vi "SonicShifter.vi"(7 "Action":T4, 8 "error in (no error)":errorcluster, 9 "Default Position":bool, 10 "Actuate?":bool, 11 "SolenoidDevRef":T1={"DevStatus"={"status"=FALSE, "code"=0, "source"=""}, "Solenoid Module"=enum."Solenoid Module 1", "Forward Solenoid Channel"=enum."Invalid", "Reverse Solenoid Channel"=enum."Invalid"}) -> (0 "error out":errorcluster)   [LabVIEW 2015]
doc: "Controls a single solenoid. It has the following actions:\n-Init: takes a reference to a single solenoid and stores it in a shift register so that the reference does not need to be passed again. Also takes a boolean for default position: if default position is false (the \"normal\" case), then Off corresponds to the retracted state and On corresponds to the actuated state. If default position is true, then Off corresponds to the *actuated* state and On corresponds to the *retracted* state.\n-SetValue: sets the position of the solenoid. True actuates the solenoid, false retracts it.\n-Disable: sets the solenoid to the retracted position."
uses:
  SingleSolenoidAction.ctl
  <vilib>/Rock Robotics/WPI/Solenoid/WPI_SolenoidDevRef.ctl
  <vilib>/Rock Robotics/SystemInterfaces/Typedef/FPGA_TypedefSolenoidModule.ctl
  <vilib>/Rock Robotics/WPI/Solenoid/WPI_SolenoidChannel.ctl
  <vilib>/Rock Robotics/WPI/Solenoid/WPI_SolenoidValue.ctl
  LEDSaction.ctl
  <vilib>/Rock Robotics/WPI/Solenoid/WPI_SolenoidSetEnum.vi
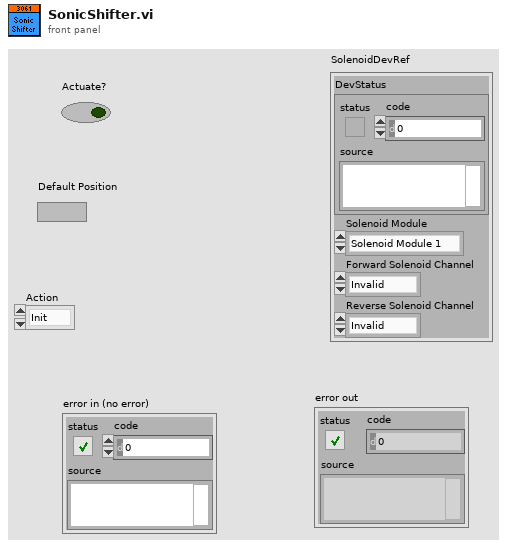
[diagram p1: front panel]
types:
  T1 = typedef "WPI_SolenoidDevRef.ctl" = cluster{"DevStatus":errorcluster, "Solenoid Module":T2, "Forward Solenoid Channel":T3, "Reverse Solenoid Channel":T3}
  T2 = typedef "FPGA_TypedefSolenoidModule.ctl" = enum16{"Solenoid Module 1", "Solenoid Module 2"}
  T3 = typedef "WPI_SolenoidChannel.ctl" = enum8{"Solenoid 1", "Solenoid 2", "Solenoid 3", "Solenoid 4", "Solenoid 5", "Solenoid 6", "Solenoid 7", "Solenoid 8", "Invalid"}
  T4 = typedef "SingleSolenoidAction.ctl" = enum16{"Init", "SetState", "Disable"}
  T5 = typedef "WPI_SolenoidValue.ctl" = enum16{"Off", "On", "Forward", "Reverse"}
  T6 = typedef "LEDSaction.ctl" = enum16{"Init", "10SecondsLeft", "LimitDown", "LimitUp", "CollectDown", "CollectUp", "NotHot", "Hot", "Shift", "RollBack", "RollFwd", "Shoot", "Distance Low", "DistanceHigh", "PressureLow", "PressureHigh"}
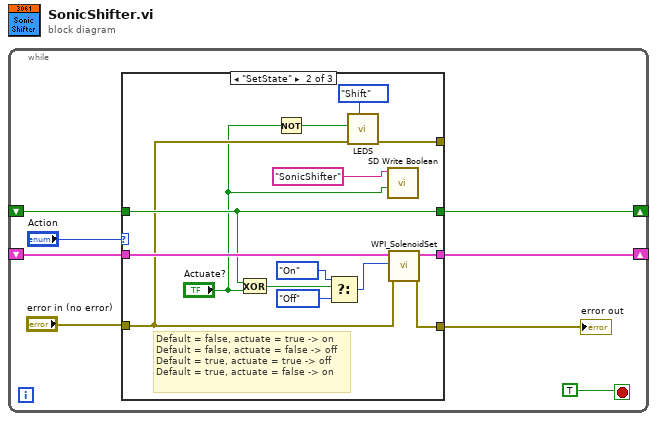
[diagram p0: block diagram]
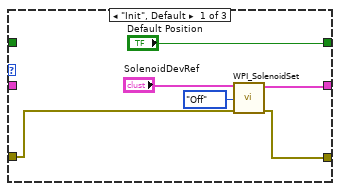
[diagram p2: hidden frame]
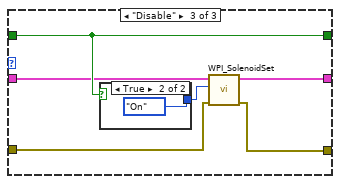
[diagram p3: hidden frame]
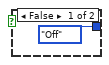
[diagram p4: hidden frame]
diagram:
  n1 = while {
    shift-right: [w6] -> _
    shift-left: _ -> [w8]
    shift-right: [w4] -> _
    shift-left: _ -> [w3]
    stop <- TRUE stop-if-true
    n2 = case shown="\"SetState\"" "Action" {
      tunnel: w8 -> [_ w21 w33]
      tunnel: ["Default Position" w21 w33] -> w6
      tunnel: [w12 w27 w31] -> w4
      tunnel: w3 -> [_ w28 w32]
      tunnel: "error in (no error)" -> [w11 w19 w30]
      tunnel: [w10 w26 w29] -> w1
      tunnel: [_ w18 _] -> _
      frame "Init", Default {
        n3 = call-poly <vilib>:"WPI_SolenoidSet.vi"("error in (no error)"=w11, "Value"=WPI_SolenoidValue."Off", "SolenoidDevRef"="SolenoidDevRef") -> ("error out"=w10:errorcluster, "SolenoidDevRef"=w12:T1)  [unwired: 7 in]
      }
      frame "SetState" {
        # "Default = false, actuate = true -> on\nDefault = false, actuate = false -> off\nDefault = true, actuate = true -> off\nDefault = true, actuate = false -> on"
        n4 = Exclusive Or(1:"Actuate?", 2:w21) -> (0:w23:bool)
        n5 = Not(x="Actuate?") -> (.not. x?=w17:bool)
        n6 = Select(t=WPI_SolenoidValue."On" ("Value"), s=w23, f=WPI_SolenoidValue."Off" ("Value")) -> (s? t:f=w22:T5)
        n7 = call "LEDS.vi"("Action"=LEDSaction."Shift", "error in"=w19, "On/Off"=w17) -> ("error out"=w18:errorcluster)  [unwired: 8 in]
        n8 = call <vilib>:"SD Write Boolean.vi"("Boolean"="Actuate?", "Name"="SonicShifter") -> ()  [unwired: 8 in, 2 out]
        n9 = call-poly <vilib>:"WPI_SolenoidSet.vi"("error in (no error)"=w19, "Value"=w22, "SolenoidDevRef"=w28) -> ("error out"=w26:errorcluster, "SolenoidDevRef"=w27:T1)  [unwired: 7 in]
      }
      frame "Disable" {
        n10 = case shown="True" w33 {
          tunnel: [WPI_SolenoidValue."Off" ("Value") WPI_SolenoidValue."On" ("Value")] -> w34
          frame False {
          }
          frame True {
          }
        }
        n11 = call-poly <vilib>:"WPI_SolenoidSet.vi"("error in (no error)"=w30, "Value"=w34, "SolenoidDevRef"=w32) -> ("error out"=w29:errorcluster, "SolenoidDevRef"=w31:T1)  [unwired: 7 in]
      }
    }
    "error out" <- w1
  }
